vi "Write Optional Plane Plane Type.vi"(8 "error in (no error)":errorcluster, 10 "PlaneType":T1(ring), 11 "XYGraph.lvclass in":refnum<class "XYGraph.lvclass">) -> (0 "error out":errorcluster, 3 "XYGraph.lvclass out":refnum<class "XYGraph.lvclass">)   [LabVIEW 2015, in "XYGraph.lvclass"]
uses:
  XYGraph.lvclass
  XYGraph.lvclass/XYGraph.ctl
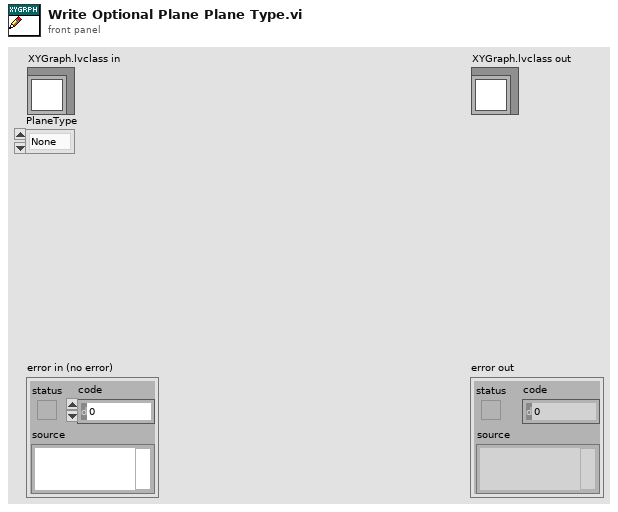
[diagram p1: front panel]
types:
  T1 = enum16{"None", "Nyquist", "Nichols", "S Plane", "Z Plane"}
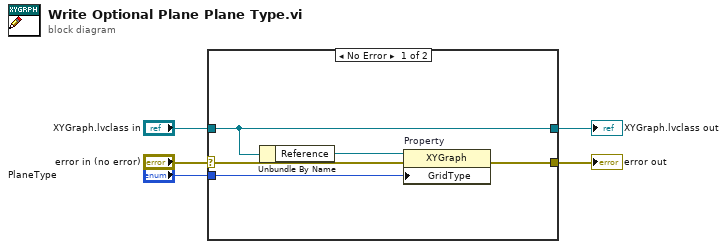
[diagram p0: block diagram]
diagram:
  n1 = case shown="No Error" "error in (no error)" {
    selector: "error in (no error)" -> [w6 w12]
    tunnel: [w10 w12] -> w4
    tunnel: [w8 w11] -> w2
    tunnel: "XYGraph.lvclass in" -> [w8 w11]
    tunnel: "PlaneType" -> [w9 _]
    frame No Error {
      n2 = Unbundle By Name(w8) -> ("Reference"=w7:refnum<vi>)
      n3 = property on="Property" class="XYGraph"(reference=w7, error in=w6, "GridType"=w9) -> (error out=w10:errorcluster)  [unwired: 1 out]
    }
    frame Error {
    }
  }
  "error out" <- w4
  "XYGraph.lvclass out" <- w2
